vi "PCert-Container-CloseDB.vi"(8 "error in (no error)":errorcluster, 11 "ERP-Container-UI in":refnum<class "PCert-Container-UI.lvclass">) -> (0 "error out":errorcluster, 3 "ERP-Container-UI out":refnum<class "PCert-Container-UI.lvclass">)   [LabVIEW 2013, in "PCert-Container-UI.lvclass"]
uses:
  PCert-Container-UI.lvclass
  PCert-Container-UI.lvclass/PCert-Container-UI.ctl
  ftw-dataflow/Core/src/Database/FTW-SQLite-Connector.lvclass
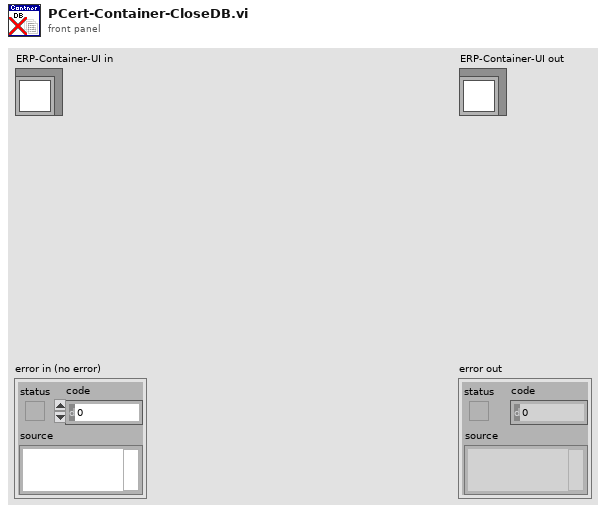
[diagram p1: front panel]
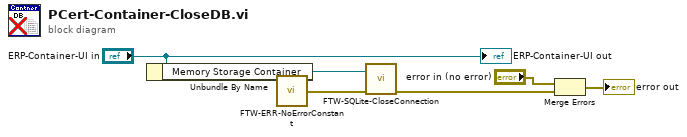
[diagram p0: block diagram]
diagram:
  n1 = Unbundle By Name("ERP-Container-UI in") -> ("Memory Storage Container"=w5:refnum<class "FTW-SQLite-Connector.lvclass">)
  n2 = call "FTW-ERR-NoErrorConstant.vi"() -> ("no error"=w4:errorcluster)
  n3 = call "FTW-SQLite-CloseConnection.vi"("SQLite Connector"=w5, "error in"=w4) -> ("error out"=w2:errorcluster)  [unwired: 13 in]
  n4 = Merge Errors("error in (no error)", w2) -> (→"error out":errorcluster)
  "ERP-Container-UI out" <- "ERP-Container-UI in"
